vi "SetParam.vi"(8 "error in (no error)":errorcluster caption="entrée d'erreur (pas d'erreur)", 10 "roc_auc_score":T1={"average"="macro", "sample_weight"=[], "max_fpr"="None", "multi_class"="raise", "labels"=["None"]}, 11 "Roc_Auc_Score.lvclass":refnum<class "Roc_Auc_Score.lvclass">) -> (0 "error out":errorcluster caption="sortie d'erreur", 3 "Roc_Auc_Score.lvclass":refnum<class "Roc_Auc_Score.lvclass">)   [LabVIEW 2020, in "Roc_Auc_Score.lvclass"]
doc: "Set Parameters"
uses:
  Roc_Auc_Score.lvclass
  Roc_Auc_Score.lvclass/Roc_Auc_Score.ctl
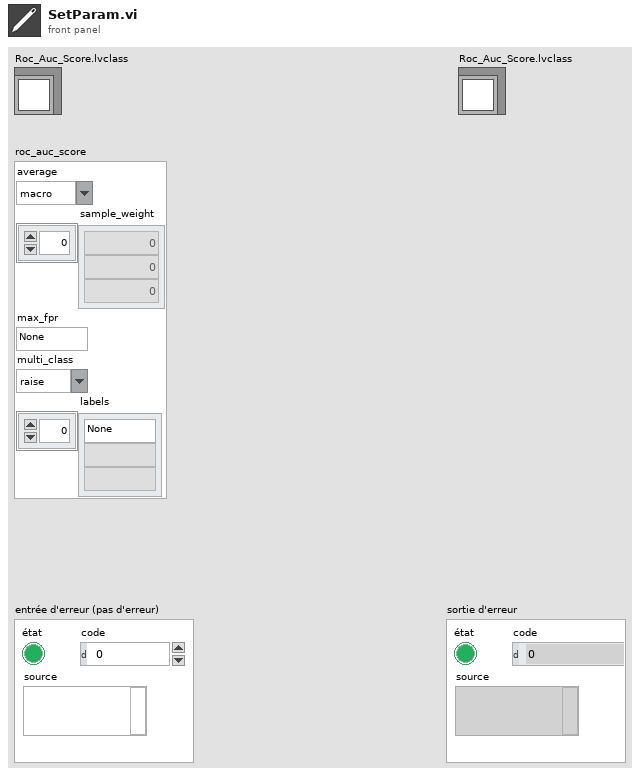
[diagram p1: front panel]
types:
  T1 = cluster{"average":string, "sample_weight":dbl[], "max_fpr":string, "multi_class":string, "labels":string[]}
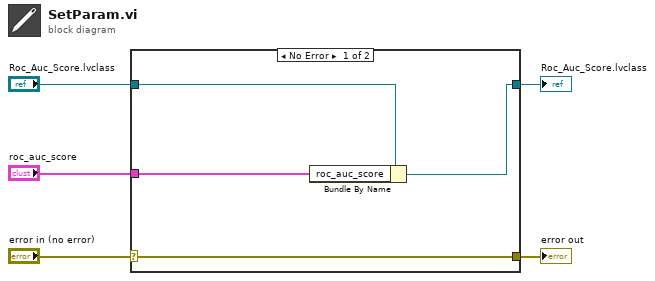
[diagram p0: block diagram]
diagram:
  n1 = case shown="No Error" "error in (no error)" {
    selector: "error in (no error)" -> [w9 w10]
    tunnel: [w9 w10] -> w4
    tunnel: [w7 w11] -> w2
    tunnel: "Roc_Auc_Score.lvclass" -> [w8 w11]
    tunnel: "roc_auc_score" -> [w6 _]
    frame No Error {
      n2 = Bundle By Name(cluster=w8, "roc_auc_score"=w6) -> (w7:refnum<class "Roc_Auc_Score.lvclass">)
    }
    frame Error {
    }
  }
  "error out" <- w4
  "Roc_Auc_Score.lvclass" <- w2
